vi "Logging_Loop.vi"(11 "TDMS DevRef In":T1) -> ()   [LabVIEW 2016]
uses:
  <vilib>/platform/TimedLoop/XDataNode/XDataNode.xnode
  <vilib>/Platform/TimedLoop/XDataNode/nitl_modes.ctl
  <vilib>/Platform/TimedLoop/XDataNode/XDNodeRunTimeDep.lvlib
  <vilib>/Platform/TimedLoop/XDataNode/wakeup.ctl
  <vilib>/Platform/TimedLoop/XDataNode/timing_clust.ctl
  <userlib>/836-Library/System/TDMS_V2/Support/Logging_Settings.ctl
  <userlib>/836-Library/System/TDMS_V2/Support/Data_To_Write.ctl
  <userlib>/836-Library/System/TDMS_V2/Support/Channel_FIFO_Config.ctl
  <userlib>/836-Library/System/TDMS_V2/Support/Group_FIFO_Config.ctl
  <userlib>/836-Library/System/TDMS_V2/Support/TDMS_DevRef.ctl
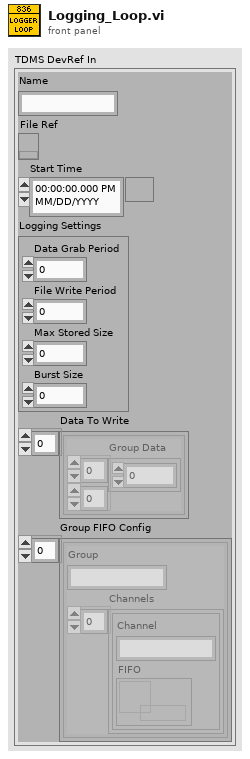
[diagram p1: front panel]
types:
  T1 = typedef "TDMS_DevRef.ctl" = cluster{"Name":string, "File Ref":refnum<k34>, "Start Time":timestamp, "Logging Settings":T2, "Data To Write":T3, "Group FIFO Config":T4[]}
  T2 = typedef "Logging_Settings.ctl" = cluster{"Data Grab Period":dbl, "File Write Period":dbl, "Max Stored Size":dbl, "Burst Size":dbl}
  T3 = typedef "Data_To_Write.ctl" = cluster{"Group Data":dbl[][]}[]
  T4 = typedef "Group_FIFO_Config.ctl" = cluster{"Group":string, "Channels":T5[]}
  T5 = typedef "Channel_FIFO_Config.ctl" = cluster{"Channel":string, "FIFO":refnum<k33>}
  T6 = typedef "XDNodeRunTimeDep.lvlib/timing_clust.ctl" = cluster{"Expected End [f-1]":u64, "Actual End [f-1]":u64, "Finished Late? [f-1]":bool, "Expected End [i-1]":u64, "Actual End [i-1]":u64, "Finished Late? [i-1]":bool, "Expected Start [i]":u64, "Actual Start [i]":u64, "Expected Start [f]":u64, "Actual Start [f]":u64, "Source Name":string, "Structure Name":string, "Period":i64, "Deadline":i64, "Offset":i64, "Start":i64, "Priority":i32, "Timeout":i32, "Mode":T7, "Wakeup Reason":T8, "Error":errorcluster, "Source Type":string, "Secondary Source Type":string, "Global End Time":u64, "Global Start Time":u64, "Frame Duration":u64, "Iteration Duration":u64, "Assigned CPU":i32, "I/O Scan Engine Mode":u32}
  T7 = typedef "XDNodeRunTimeDep.lvlib/nitl_modes.ctl" = enum32{"No Change", "Process missed periods, maintain original phase", "Discard missed periods, maintain original phase", "Process missed periods, ignore original phase", "Discard missed periods, ignore original phase"}
  T8 = typedef "XDNodeRunTimeDep.lvlib/wakeup.ctl" = enum32{"Normal", "Aborted", "Asynchronous wakeup", "Timing source error", "Timed loop error", "Timeout"}
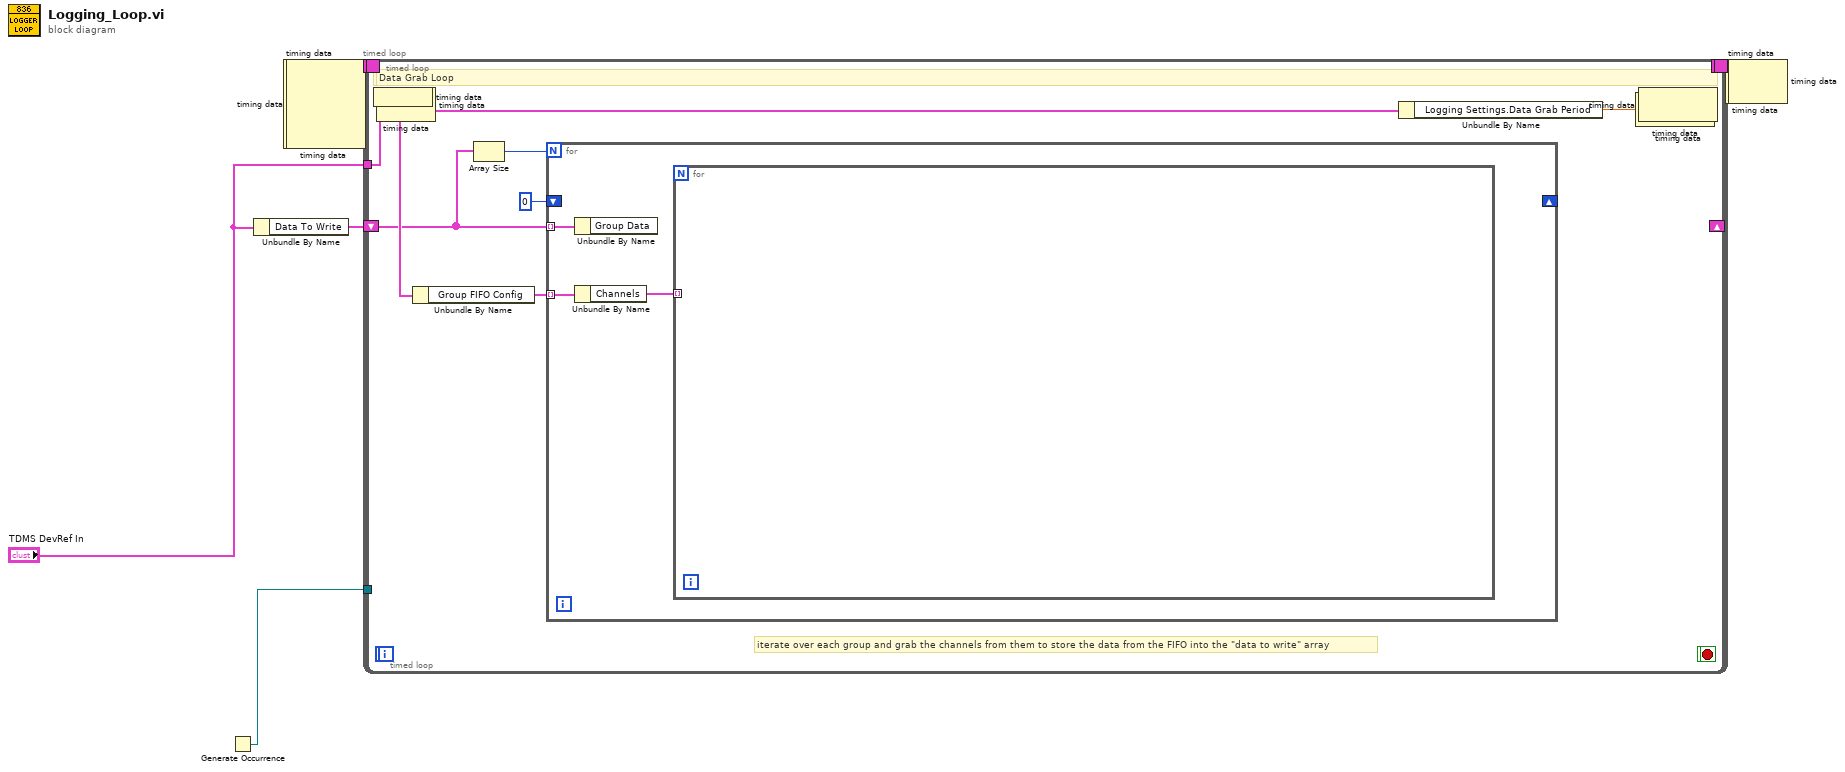
[diagram p0: block diagram]
diagram:
  n1 = Generate Occurrence() -> (w3:refnum<k4>)
  n2 = Unbundle By Name("TDMS DevRef In") -> ("Data To Write"=w2:T3)
  n3 = node-c288() -> (w5:T6)  [unwired: 4 in]
  n4 = node-c288() -> (w7:T6)  [unwired: 4 in]
  n5 = node-c288() -> (w9:T6)  [unwired: 4 in]
  n6 = timed-loop {
    timing: w5 -> [_]
    timing-out: [_] -> w4
    tunnel: w3 -> [_]
    shift-right: _ -> [_]
    shift-left: w2 -> [w10]
    tunnel: "TDMS DevRef In" -> [w12]
    stop <- _ stop-if-true
    # "iterate over each group and grab the channels from them to store the data from the FIFO into the \"data to write\" array"
    # "Data Grab Loop"
    n7 = node-c288() -> ()  [unwired: 1 in]
    n8 = Unbundle By Name(w12) -> ("Group FIFO Config"=w11:T4[])
    n9 = Array Size(array=w10) -> (size(s)=w14:i32)
    n10 = for {
      N: w14 -> [_]
      shift-right: _ -> [_]
      shift-left: 0 -> [_]
      tunnel: w11 -> [w18] mode=indexing
      tunnel: w10 -> [w16] mode=indexing
      n11 = Unbundle By Name(w16) -> ()  [unwired: 1 out]
      n12 = Unbundle By Name(w18) -> ("Channels"=w17:T5[])
      n13 = for {
        tunnel: w17 -> [_] mode=indexing
      }
    }
    n14 = Unbundle By Name(w12) -> ("Logging Settings.Data Grab Period"=w15:dbl)
    n15 = node-c288(w15) -> ()  [unwired: 1 out]
  }
  n16 = timed-loop {
    timing: w7 -> [_]
    timing-out: [_] -> w6
    stop <- _ stop-if-true
    # "Data Grab Loop"
    n17 = node-c288() -> ()  [unwired: 1 in, 1 out]
    n18 = node-c288() -> ()  [unwired: 1 in, 1 out]
  }
  n19 = timed-loop {
    timing: w9 -> [_]
    timing-out: [_] -> w8
    stop <- _ stop-if-true
    # "Data Grab Loop"
    n20 = node-c288() -> ()  [unwired: 1 in, 1 out]
    n21 = node-c288() -> ()  [unwired: 1 in, 1 out]
  }
  n22 = node-c288(w4) -> ()  [unwired: 1 out]
  n23 = node-c288(w6) -> ()  [unwired: 1 out]
  n24 = node-c288(w8) -> ()  [unwired: 1 out]
